vi "PID Tuner UDP.vi"() -> ()   [LabVIEW 2016]
panel:
  in  "Acceleration":dbl
  in  "Cruise Velocity":dbl
  in  "Reset Average":bool=TRUE
  out "Average Deviation":dbl
  out "Deviation Plot":dynamicdata(graph)=[{"t0"=timestamp(3570920707.45624 s since 1904-01-01), "dt"=1.0, "Y"=[-3600.0]}, {"t0"=timestamp(3570920707.45624 s since 1904-01-01), "dt"=1.0, "Y"=[0.0]}]
  out "Deviation":dbl=-3600.0
  in  "Setpoint":dbl=-3600.0
  in  "f":dbl=0.03
  in  "kD":dbl=10.0
  in  "kI":dbl
  in  "kP":dbl=1.0
  in  "port":u16=5809
  out "Name":string
  out "ActualValue":dbl
  out "DesiredValue":dbl=-3600.0
  out "Actual vs. Desired":dynamicdata(graph)=[{"t0"=timestamp(3570920707.45624 s since 1904-01-01), "dt"=1.0, "Y"=[0.0]}, {"t0"=timestamp(3570920707.45624 s since 1904-01-01), "dt"=1.0, "Y"=[-3600.0]}]
  # ".32"
  # ".00026"
  # "18"
  # ".076"
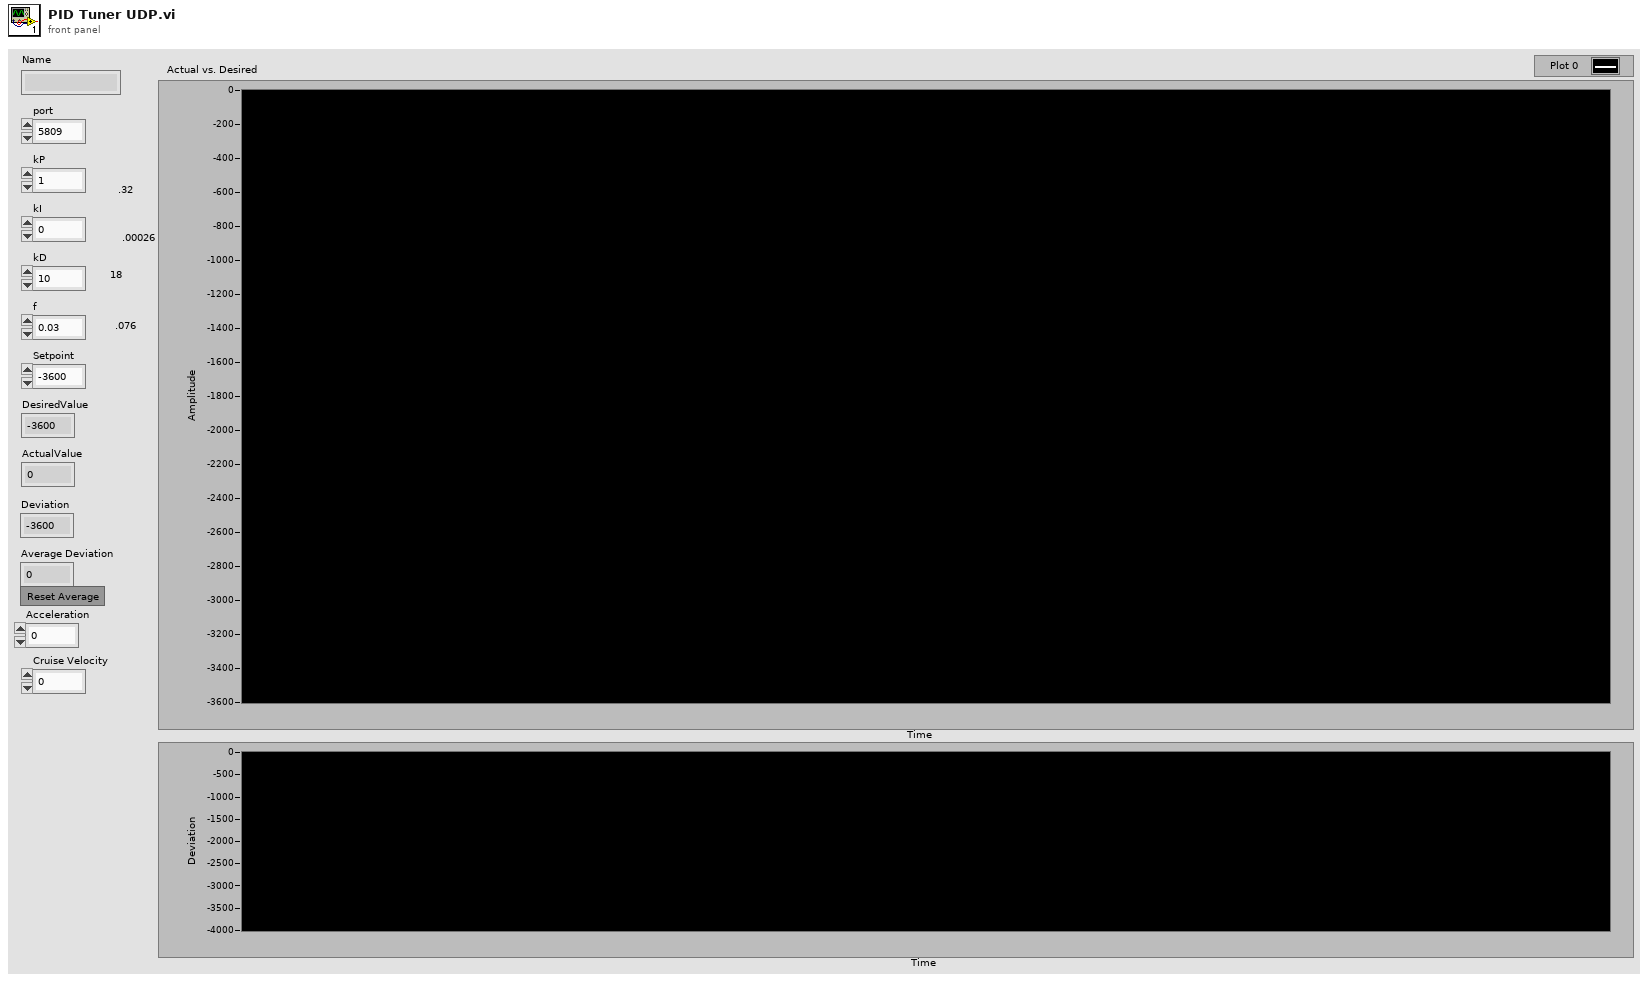
[diagram p1: front panel]
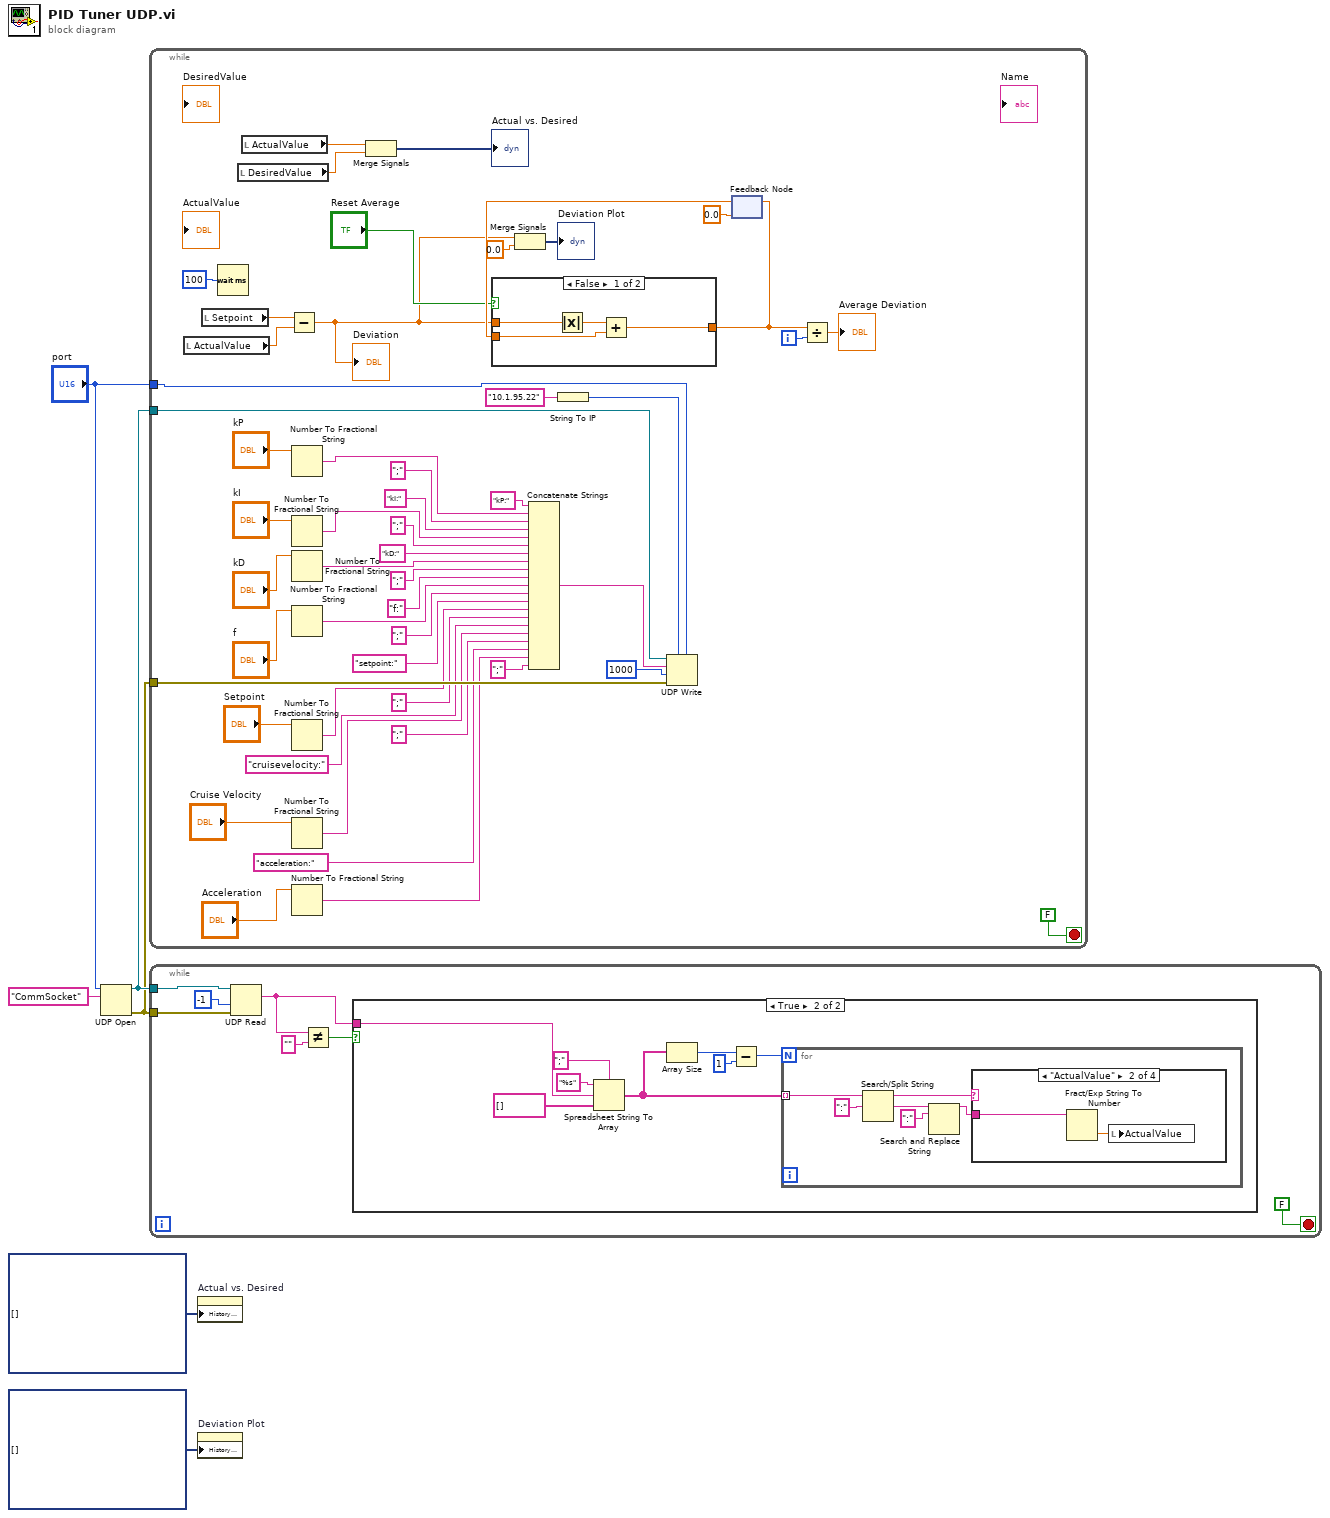
[diagram p0: block diagram]
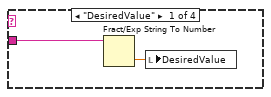
[diagram p3: hidden frame]
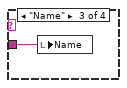
[diagram p4: hidden frame]
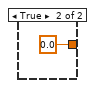
[diagram p6: hidden frame]
diagram:
  n1 = UDP Open(10:"CommSocket" ("service name"), 11:"port") -> (port=w4:refnum<k16>, 0:w3:errorcluster)  [unwired: 3 in, 1 out]
  n2 = while {
    tunnel: w4 -> [w54]
    tunnel: w3 -> [w53]
    tunnel: "port" -> [w51]
    i -> [w20]
    stop <- FALSE stop-if-true
    n3 = local read "ActualValue"() -> (w24:dbl)
    n4 = local read "Setpoint"() -> (w25:dbl)
    n5 = Wait (ms)(milliseconds to wait=u32 100) -> ()  [unwired: 1 out]
    n6 = local read "DesiredValue"() -> (w56:dbl)
    n7 = local read "ActualValue"() -> (w57:dbl)
    n8 = Subtract(x=w25, y=w24) -> (x-y=w17:dbl)
    "Deviation" <- w17
    n9 = Number To Fractional String(number="kP") -> (F-format string=w48:string)  [unwired: 3 in]
    n10 = Number To Fractional String(number="kI") -> (F-format string=w44:string)  [unwired: 3 in]
    n11 = Number To Fractional String(number="kD") -> (F-format string=w41:string)  [unwired: 3 in]
    n12 = Number To Fractional String(number="f") -> (F-format string=w38:string)  [unwired: 3 in]
    n13 = Number To Fractional String(number="Setpoint") -> (F-format string=w28:string)  [unwired: 3 in]
    n14 = Number To Fractional String(number="Cruise Velocity") -> (F-format string=w12:string)  [unwired: 3 in]
    n15 = Number To Fractional String(number="Acceleration") -> (F-format string=w8:string)  [unwired: 3 in]
    n16 = Merge Signals(w57, w56) -> (→"Actual vs. Desired":dynamicdata)
    n17 = Merge Signals(w17, 0.0) -> (→"Deviation Plot":dynamicdata)
    n18 = Concatenate Strings("kP:", w48, ";", "kI:", w44, ";", "kD:", w41, ";", "f:", w38, ";", "setpoint:", w28, ";", "cruisevelocity:", w12, ";", "acceleration:", w8, ";") -> (w32:string)
    n19 = String To IP(1:"10.1.95.22" ("name")) -> (0:w52:u32)
    n20 = UDP Write(address=w52, port or service name=w51, connection ID=w54, data in=w32, 8:w53, 9:1000 ("timeout ms (25000)")) -> ()  [unwired: 2 out]
    n21 = feedback #1(0.0) -> (w23:dbl)
    n22 = case shown="False" "Reset Average" {
      tunnel: w17 -> [w61 _]
      tunnel: w23 -> [w60 _]
      tunnel: [w59 0.0] -> w21
      frame False {
        n23 = Absolute Value(x=w61) -> (abs(x)=w58:dbl)
        n24 = Add(x=w58, y=w60) -> (x+y=w59:dbl)
      }
      frame True {
      }
    }
    n25 = feedback-in #1(w21) -> ()
    n26 = Divide(x=w21, y=w20) -> (x/y=→"Average Deviation":dbl)
  }
  n27 = while {
    tunnel: w4 -> [w65]
    tunnel: w3 -> [w64]
    stop <- FALSE stop-if-true
    n28 = UDP Read(connection ID=w65, timeout ms (25000)=-1, 8:w64) -> (data out=w69:string)  [unwired: 1 in, 4 out]
    n29 = Not Equal?(x=w69, y="") -> (x != y?=w68:bool)
    n30 = case shown="True" w68 {
      tunnel: w69 -> [_ w77]
      frame False {
      }
      frame True {
        n31 = Spreadsheet String To Array(delimiter (Tab)=";" ("search string/char (-)"), format string="%s", spreadsheet string=w77, array type (2D Dbl)=string[] []) -> (array=w73:string[])
        n32 = Array Size(array=w73) -> (size(s)=w72:i32)
        n33 = Subtract(x=w72, y=1) -> (x-y=w70:i32)
        n34 = for {
          N: w70 -> [_]
          tunnel: w73 -> [w83] mode=indexing
          n35 = Search/Split String(string=w83, search string/char (-)=":") -> (substring before match=w81:string, match + rest of string=w80:string)  [unwired: 1 in, 1 out]
          n36 = Search and Replace String(input string=w80, search string=":" ("replace string (\"\")")) -> (result string=w78:string)  [unwired: 6 in, 3 out]
          n37 = case shown="\"ActualValue\"" w81 {
            tunnel: w78 -> [w85 w87 w88 _]
            frame "DesiredValue" {
              n38 = Fract/Exp String To Number(string=w85) -> (number=w84:dbl)  [unwired: 3 in, 1 out]
              n39 = local write "DesiredValue"(w84) -> ()
            }
            frame "ActualValue" {
              n40 = Fract/Exp String To Number(string=w87) -> (number=w86:dbl)  [unwired: 3 in, 1 out]
              n41 = local write "ActualValue"(w86) -> ()
            }
            frame "Name" {
              n42 = local write "Name"(w88) -> ()
            }
            frame "False", Default {
            }
          }
        }
      }
    }
  }
  n43 = property on="Actual vs. Desired" class="WFChart (strict)"("History Data"=dynamicdata[] []) -> ()  [unwired: 2 in, 2 out]
  n44 = property on="Deviation Plot" class="WFChart (strict)"("History Data"=dynamicdata[] []) -> ()  [unwired: 2 in, 2 out]
